vi "Get ErrorHandlerPPL Version Number.vi"(8 "Error In":errorcluster) -> (0 "Error Out":errorcluster, 3 "ErrorHandlerPPL Version Number":string)   [LabVIEW 2023, in "Error Manager.lvlib"]
doc: "This VI:\n1. When owned by (build into) a PPL: returns the version number of the PPL, for example 1.0.0.0 or 5.6.7.8\n2. When not owned by a PPL: returns \"<LabVIEW Dev Environment>\"\n\nPPL = LabVIEW Packed Project Library (.lvlibp file extension)"
uses:
  Error Manager.lvlib
  <vilib>/Utility/LVLibp/NI_PackedLibraryUtility.lvlib
panel:
  out "TRUE = this VI is owned by a PPL":bool
  out "Owner PPL Filepath":path
  # "Development\nControls or indicators that are useful for development or testing, but which are not outputs of the VI."
  # "Input\nInputs to the VI"
  # "Output\nOutputs of the VI"
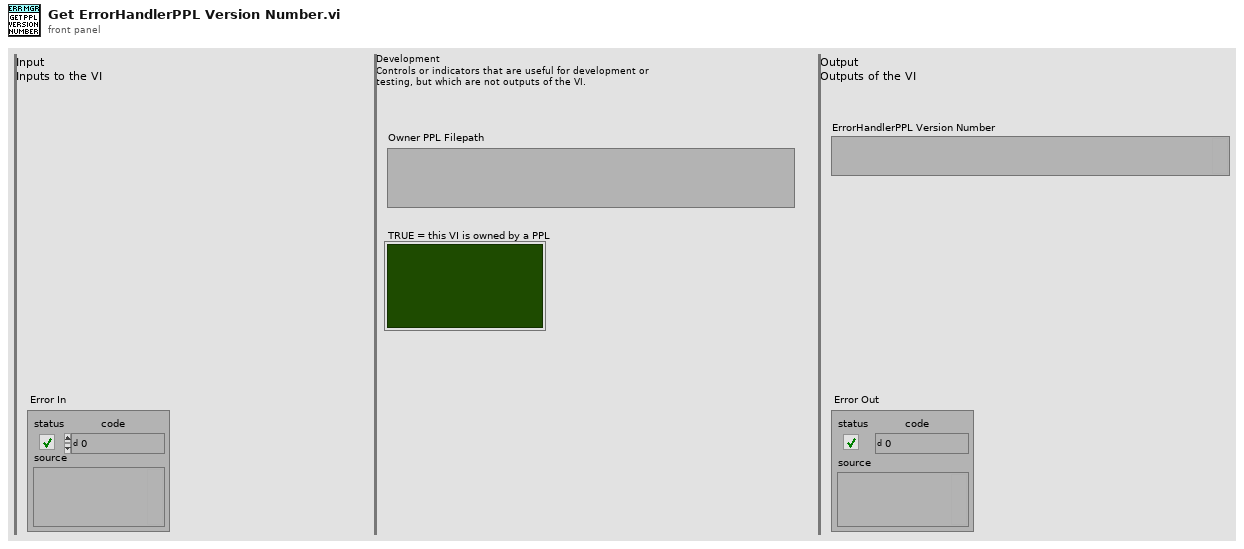
[diagram p1: front panel]
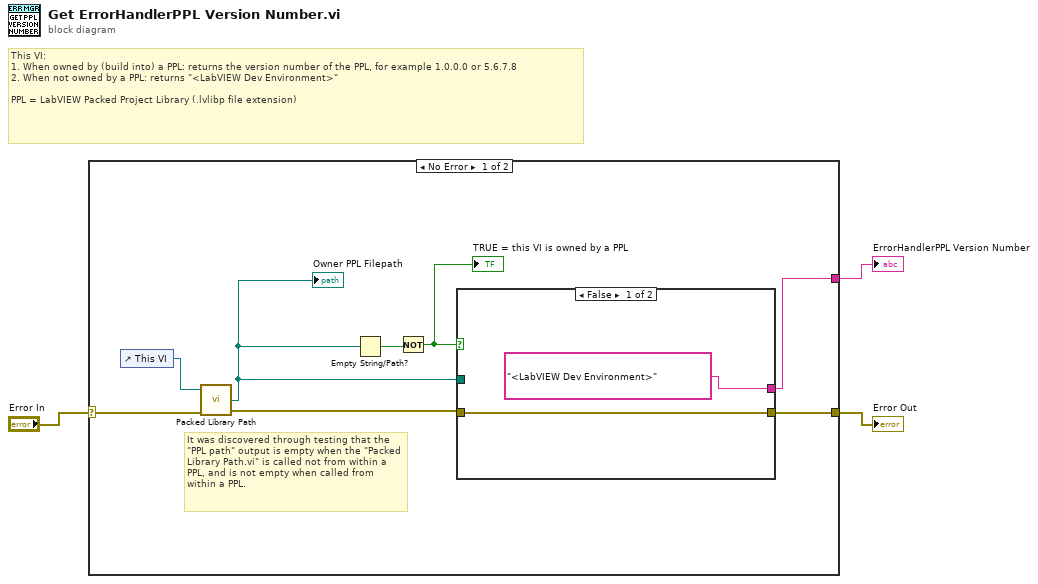
[diagram p0: block diagram]
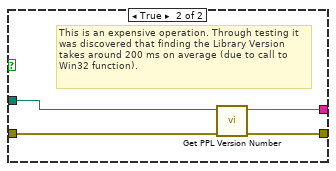
[diagram p2: hidden frame]
diagram:
  # "This VI:\n1. When owned by (build into) a PPL: returns the version number of the PPL, for example 1.0.0.0 or 5.6.7.8\n2. When not owned by a PPL: returns \"<LabVIEW Dev Environment>\"\n\nPPL = LabVIEW Packed Project Library (.lvlibp file extension)"
  n1 = case shown="No Error" "Error In" {
    selector: "Error In" -> [w10 w18]
    tunnel: [w9 w18] -> w2
    tunnel: [w11 _] -> w1
    frame No Error {
      # "It was discovered through testing that the \"PPL path\" output is empty when the \"Packed Library Path.vi\" is called not from within a PPL, and is not empty when called from within a PPL."
      n2 = control-ref of="This VI"() -> (w8:refnum<vi>)
      n3 = call <vilib>:"Packed Library Path.vi"("error in (no error)"=w10, "vi reference"=w8) -> ("error out"=w7:errorcluster, "packed library path"=w4:path)  [unwired: 1 in, 1 out]
      "Owner PPL Filepath" <- w4
      n4 = Empty String/Path?(string/path=w4) -> (empty?=w6:bool)
      n5 = Not(x=w6) -> (.not. x?=w5:bool)
      "TRUE = this VI is owned by a PPL" <- w5
      n6 = case shown="False" w5 {
        tunnel: [w13 w17] -> w9
        tunnel: ["<LabVIEW Dev Environment>" ("result string") w16] -> w11
        tunnel: w7 -> [w13 w15]
        tunnel: w4 -> [_ w14]
        frame False {
        }
        frame True {
          # "This is an expensive operation. Through testing it was discovered that finding the Library Version takes around 200 ms on average (due to call to Win32 function)."
          n7 = call "Get PPL Version Number.vi"("error in"=w15, "EXE Filepath"=w14) -> ("error out"=w17:errorcluster, "PPL Version Number"=w16:string)  [unwired: 8 in]
        }
      }
    }
    frame Error {
    }
  }
  "Error Out" <- w2
  "ErrorHandlerPPL Version Number" <- w1
